vi "Median_Filtering.vi"(6 "Feedback Array":dbl[](array[numeric]), 7 "N":i32=10, 10 "CurrentValue":dbl) -> (2 "Median Value":dbl, 4 "Array to Back Feed":dbl[](array[numeric]))   [LabVIEW 2019]
panel:
  out "sorted array":dbl[](array[numeric])
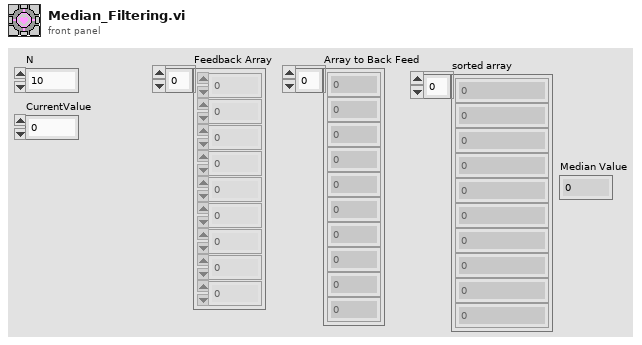
[diagram p1: front panel]
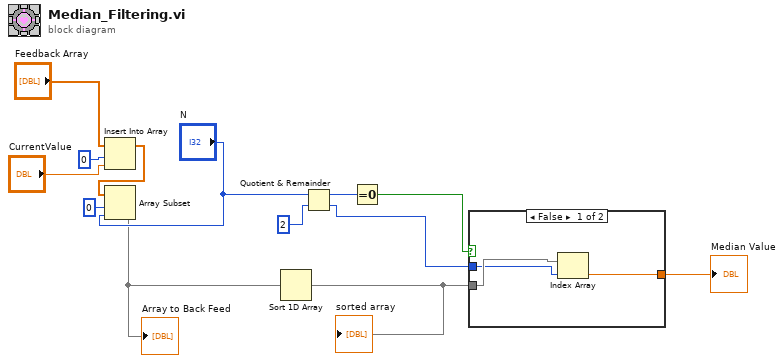
[diagram p0: block diagram]
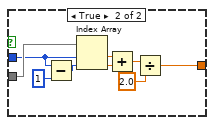
[diagram p2: hidden frame]
diagram:
  n1 = Insert Into Array(array="Feedback Array", index=0, new element="CurrentValue") -> (w3:dbl[])
  n2 = Array Subset(array=w3, index=0, length="N") -> (w2:dbl[])
  "Array to Back Feed" <- w2
  n3 = Sort 1D Array(array=w2) -> (sorted array=w9:dbl[])
  "sorted array" <- w9
  n4 = Quotient & Remainder(x="N", y=2) -> (x-y*floor(x/y)=w12:i32, floor(x/y)=w10:i32)
  n5 = Equal To 0?(x=w12) -> (x = 0?=w11:bool)
  n6 = case shown="False" w11 {
    tunnel: w10 -> [w14 w22]
    tunnel: w9 -> [w16 w25]
    tunnel: [w15 w17] -> w7
    frame False {
      n7 = Index Array(array=w16, index=w14) -> (element=w15:dbl)
    }
    frame True {
      n8 = Subtract(x=w22, y=1) -> (x-y=w23:i32)
      n9 = Index Array(array=w25, index #1=w22, index #2=w23) -> (element #1=w20:dbl, element #2=w21:dbl)
      n10 = Add(x=w20, y=w21) -> (x+y=w19:dbl)
      n11 = Divide(x=w19, y=2.0) -> (x/y=w17:dbl)
    }
  }
  "Median Value" <- w7
